vi "SendMotionMovingBool.vi"(8 "error in (no error)":errorcluster, 9 "Axis True= Moving":bool, 10 "mmWave Axis Name":string, 11 "SendMessage in":refnum<class "SendMessage.lvclass">) -> (0 "error out":errorcluster, 3 "SendMessage out":refnum<class "SendMessage.lvclass">)   [LabVIEW 2019, in "SendMessage.lvclass"]
uses:
  SendMessage.lvclass
  Support/MessageAPI/UIMessage.ctl
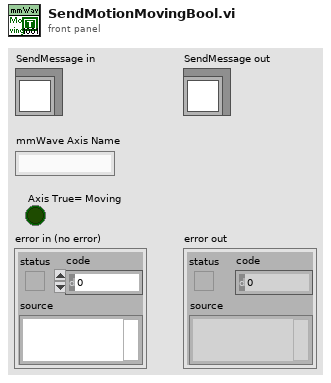
[diagram p1: front panel]
types:
  T1 = typedef "UIMessage.ctl" = cluster{"EventCode":i32, "Numeric":dbl, "String":string, "Variant":variant}
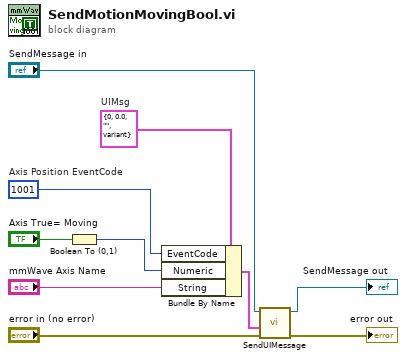
[diagram p0: block diagram]
diagram:
  w4 = T1 {"EventCode"=0, "Numeric"=0.0, "String"="", "Variant"=variant}  # UIMsg
  w2 = 1001  # Axis Position EventCode
  n1 = Boolean To (0,1)(Boolean="Axis True= Moving") -> (0, 1=w1:i16)
  n2 = Bundle By Name(cluster=w4, "EventCode"=w2, "Numeric"=w1, "String"="mmWave Axis Name") -> (w3:T1)
  n3 = call-dynamic "SendUIMessage.vi"("error in (no error)"="error in (no error)", "UIMsg"=w3, "SendMessage in"="SendMessage in") -> ("error out"=→"error out":errorcluster, "SendMessage out"=→"SendMessage out":refnum<class "SendMessage.lvclass">)  [unwired: 7 in]
